vi "Count.vi"(3 "MsgPackMap in":refnum<class "MsgPackMap.lvclass">) -> (1 "Count":u64)   [LabVIEW 2020, in "MessagePack.lvlib" / "MsgPackMap.lvclass"]
uses:
  MsgPackMap.lvclass
  MsgPackMap.lvclass/MsgPackMap.ctl
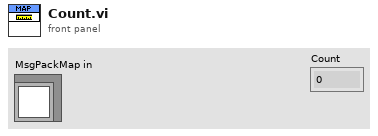
[diagram p1: front panel]
types:
  T1 = map{refnum<class "IMessagePackObject.lvclass">, refnum<class "IMessagePackObject.lvclass">}
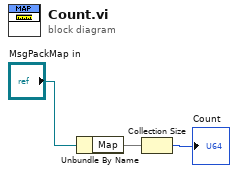
[diagram p0: block diagram]
diagram:
  n1 = Unbundle By Name("MsgPackMap in") -> ("Map"=w2:T1)
  n2 = Collection Size(1:w2) -> (0:→"Count":i32)
